vi "util_GetFilterWheelPosition.vi"(2 "Position (Simulate)":i32, 3 "Filter Wheel":enum16{"473nm", "532nm"}(ring)) -> (0 "Filter Transmission":dbl, 1 "Filter Position":i32)   [LabVIEW 2012]
uses:
  <vilib>/Utility/error.llb/DialogType.ctl
  <vilib>/Utility/error.llb/Error Cluster From Error Code.vi
  <vilib>/ErrorRing/Error Ring.xnode
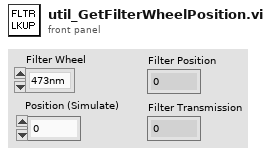
[diagram p1: front panel]
types:
  T1 = typedef "DialogType.ctl" = u16
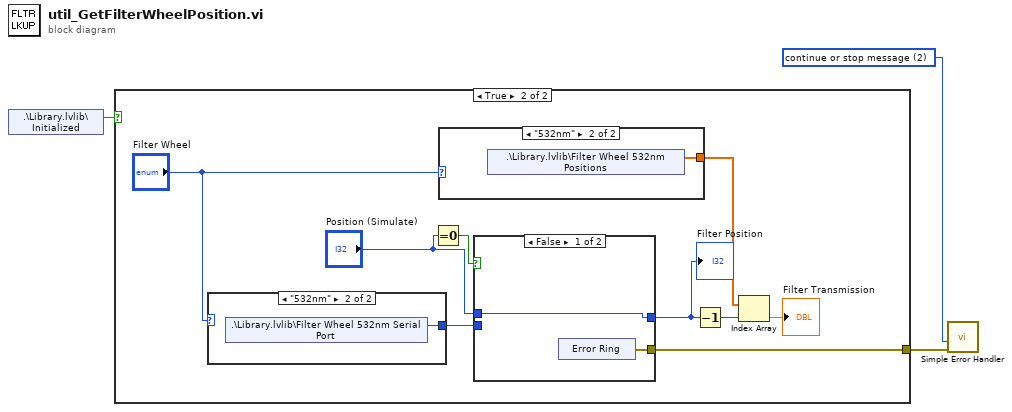
[diagram p0: block diagram]
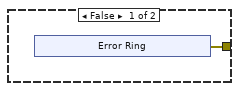
[diagram p2: hidden frame]
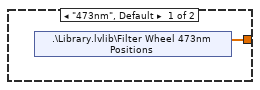
[diagram p3: hidden frame]
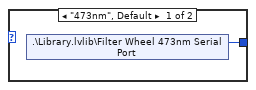
[diagram p4: hidden frame]
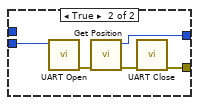
[diagram p5: hidden frame]
diagram:
  w2 = T1 2 items=["no dialog", "OK message", "continue or stop message", "OK message + warnings", "continue/stop + warnings"] ("type of dialog (OK msg:1)")
  n1 = shared-variable ".\\Library.lvlib\\Initialized"() -> (w3:bool)  [unwired: 1 in, 1 out]
  n2 = case shown="True" w3 {
    tunnel: [w4 w10] -> w1
    frame False {
      n3 = xnode "Error Ring"() -> ("error out"=w4:errorcluster)
    }
    frame True {
      n4 = case shown="\"532nm\"" "Filter Wheel" {
        tunnel: [w21 w22] -> w16
        frame "473nm", Default {
          n5 = shared-variable ".\\Library.lvlib\\Filter Wheel 473nm Serial Port"() -> (w21:i8)  [unwired: 1 in, 1 out]
        }
        frame "532nm" {
          n6 = shared-variable ".\\Library.lvlib\\Filter Wheel 532nm Serial Port"() -> (w22:i8)  [unwired: 1 in, 1 out]
        }
      }
      n7 = Equal To 0?(x="Position (Simulate)") -> (x = 0?=w18:bool)
      n8 = case shown="\"532nm\"" "Filter Wheel" {
        tunnel: [w19 w20] -> w11
        frame "473nm", Default {
          n9 = shared-variable ".\\Library.lvlib\\Filter Wheel 473nm Positions"() -> (w19:dbl[])  [unwired: 1 in, 1 out]
        }
        frame "532nm" {
          n10 = shared-variable ".\\Library.lvlib\\Filter Wheel 532nm Positions"() -> (w20:dbl[])  [unwired: 1 in, 1 out]
        }
      }
      n11 = case shown="False" w18 {
        tunnel: [w24 w28] -> w15
        tunnel: "Position (Simulate)" -> [w24 _]
        tunnel: w16 -> [_ w27]
        tunnel: [w23 w26] -> w10
        frame False {
          n12 = xnode "Error Ring"() -> ("error out"=w23:errorcluster)
        }
        frame True {
          n13 = call "UART Open.vi"("Serial Port"=w27) -> ("error out"=w30:errorcluster)  [unwired: 9 in, 1 out]
          n14 = call "Get Position.vi"("error in (no error)"=w30) -> ("error out"=w29:errorcluster, "Position"=w28:i32)  [unwired: 9 in]
          n15 = call "UART Close.vi"("error in (no error)"=w29) -> ("error out"=w26:errorcluster)  [unwired: 10 in]
        }
      }
      "Filter Position" <- w15
      n16 = Decrement(x=w15) -> (x-1=w14:i32)
      n17 = Index Array(array=w11, index=w14) -> (element=→"Filter Transmission":dbl)
    }
  }
  n18 = call <vilib>:"Simple Error Handler.vi"("type of dialog (OK msg:1)"=w2, "error in (no error)"=w1) -> ()  [unwired: 3 in, 5 out]
